vi "WaitPassTacticCheckStateChange.vi"(4 "Tactic index in":i32, 6 "Role ofRobotThat\nmake the pass":T1=enum."PassKicker", 8 "error in (no error)":errorcluster, 9 "Robot in":refnum<class "Robot.lvclass">, 10 "Game":refnum<class "Game.lvclass">, 11 "WaitPassTactic in":refnum<class "WaitPassTactic.lvclass">) -> (0 "error out":errorcluster, 2 "States":enum16{"State 0", "State 1", "State 2", "Exit"}(ring), 3 "WaitPassTactic out":refnum<class "WaitPassTactic.lvclass">)   [LabVIEW 2023, in "WaitPassTactic.lvclass"]
uses:
  WaitPassTactic.lvclass
  Game_class/Game.lvclass
  Robot_class/roles.ctl
  Robot_class/Robot.lvclass
  Game_class/Game.lvclass/Game.ctl
  Team_class/Team.lvclass/Team.ctl
  Robot_class/Robot.lvclass/Robot.ctl
  Robot_class/Read role.vi
  Game_class/Read OffensiveTeam.vi
  Game_class/Read Utilities.lvclass.vi
  Game_class/Read BallRef.vi
  Team_class/Read RobotRef.vi
  Ally_class/Ally.lvclass
  Utilities_class/Utilities.lvclass
  Ball_class/Ball.lvclass
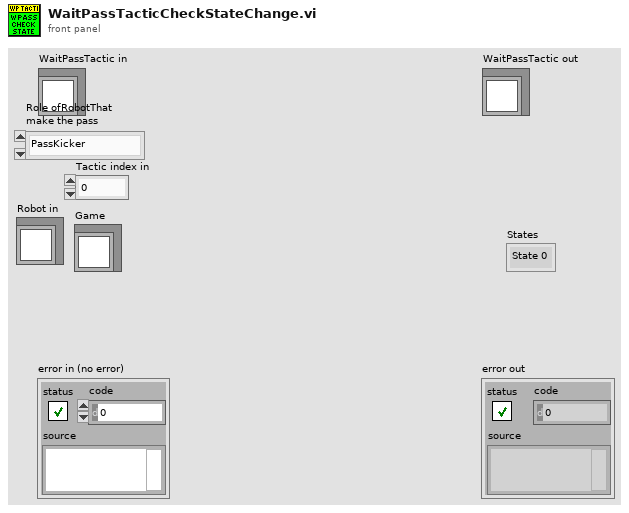
[diagram p1: front panel]
types:
  T1 = typedef "roles.ctl" = enum16{"BallChallengerAttackerVSS", "NormalAttackerVSS", "AttackerAimGoalVSS", "DefenderAreaVSS", "KeeperVSS", "Tabler", "TableFinalizer", "PrepareRollToPassRoller", "PrepareRollToPassReceiver", "SimplePassRoll", "SimplePassRollReceiver", "PenaltyDefense", "PreparePassReceiver 2", "PreparePassReceiver 1", "PassObserver", "Timeout", "Goto", "ZigZag", "None", "BallOutOfField", "DefenderArea", "Duelist", "AttackerStop", "FollowAttacker", "KeeperRole", "KickPenalty", "AttackerAimGoal", "AttackerBlock", "Marker", "Halt", "Shoot", "PassKicker", "PassReceiver", "TestRole", "PenaltyAttacker"}
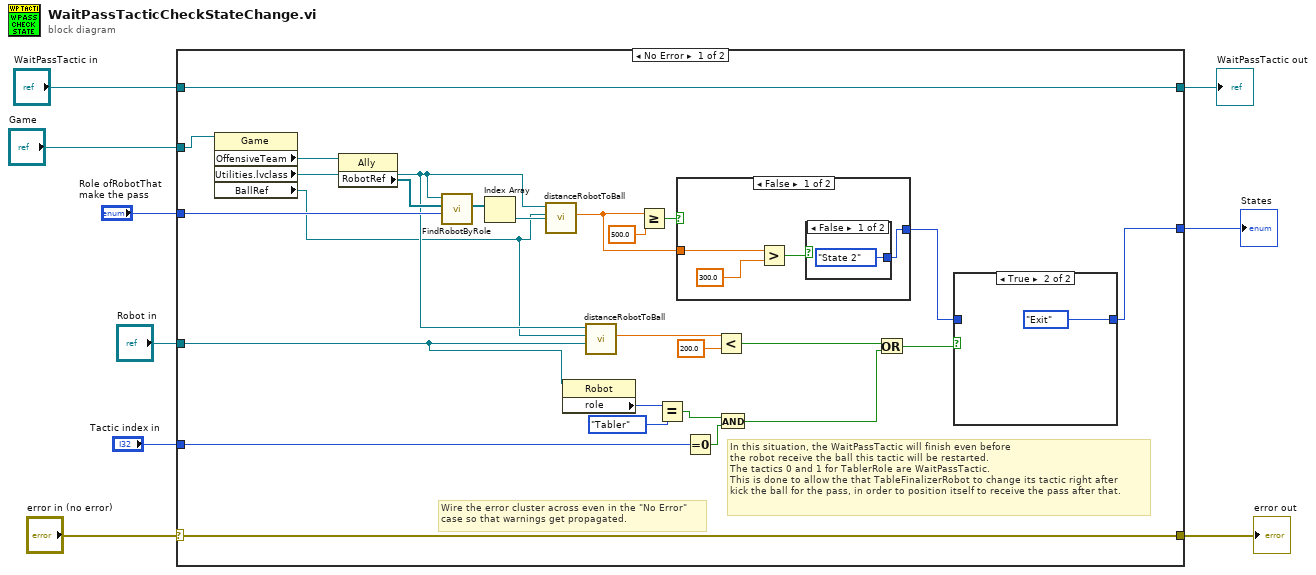
[diagram p0: block diagram]
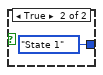
[diagram p3: hidden frame]
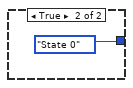
[diagram p4: hidden frame]
diagram:
  n1 = case shown="No Error" "error in (no error)" {
    selector: "error in (no error)" -> [w35 w46]
    tunnel: [w35 w46] -> w8
    tunnel: [w34 w45] -> w6
    tunnel: "WaitPassTactic in" -> [w34 w45]
    tunnel: [w22 _] -> w4
    tunnel: "Game" -> [w26 _]
    tunnel: "Role ofRobotThat\nmake the pass" -> [w21 _]
    tunnel: "Robot in" -> [w17 _]
    tunnel: "Tactic index in" -> [w12 _]
    frame No Error {
      # "In this situation, the WaitPassTactic will finish even before\nthe robot receive the ball this tactic will be restarted. \nThe tactics 0 and 1 for TablerRole are WaitPassTactic.\nThis is done to allow the that TableFinalizerRobot to change its tactic right after\nkick the ball for the pass, in order to position itself to receive the pass after that."
      # "Wire the error cluster across even in the \"No Error\"\ncase so that warnings get propagated."
      n2 = property class="Game"(reference=w26) -> ("OffensiveTeam"=w33:refnum<class "Ally.lvclass">, "Utilities.lvclass"=w20:refnum<class "Utilities.lvclass">, "BallRef"=w10:refnum<class "Ball.lvclass">)  [unwired: 1 in, 2 out]
      n3 = property class="Ally"(reference=w33) -> ("RobotRef"=w27:refnum<class "Robot.lvclass">[])  [unwired: 1 in, 2 out]
      n4 = call "FindRobotByRole.vi"("role"=w21, "RobotRef"=w27, "Utilities in"=w20) -> ("Robots"=w30:refnum<class "Robot.lvclass">[])  [unwired: 6 in, 2 out]
      n5 = Index Array(array=w30) -> (element=w29:refnum<class "Robot.lvclass">)  [unwired: 1 in]
      n6 = call "distanceRobotToBall.vi"("Robot"=w29, "Ball"=w10, "Utilities in"=w20) -> ("Distance Robot To Ball"=w28:dbl)  [unwired: 6 in, 2 out]
      n7 = property class="Robot"(reference=w17) -> ("role"=w16:T1)  [unwired: 1 in, 2 out]
      n8 = call "distanceRobotToBall.vi"("Robot"=w17, "Ball"=w10, "Utilities in"=w20) -> ("Distance Robot To Ball"=w25:dbl)  [unwired: 6 in, 2 out]
      n9 = Greater Or Equal?(x=w28, y=500.0) -> (x >= y?=w31:bool)
      n10 = Equal?(x=w16, y=roles."Tabler") -> (x = y?=w14:bool)
      n11 = case shown="False" w31 {
        tunnel: [w39 enum16{"State 0", "State 1", "State 2", "Exit"}."State 0" ("States")] -> w23
        tunnel: w28 -> [w38 _]
        frame False {
          n12 = Greater?(x=w38, y=300.0) -> (0:w40:bool)
          n13 = case shown="False" w40 {
            tunnel: [enum16{"State 0", "State 1", "State 2", "Exit"}."State 2" ("States") enum16{"State 0", "State 1", "State 2", "Exit"}."State 1" ("States")] -> w39
            frame False {
            }
            frame True {
            }
          }
        }
        frame True {
        }
      }
      n14 = Equal To 0?(x=w12) -> (x = 0?=w13:bool)
      n15 = Less?(x=w25, y=200.0) -> (x < y?=w18:bool)
      n16 = And(x=w14, y=w13) -> (x .and. y?=w11:bool)
      n17 = Or(x=w18, y=w11) -> (x .or. y?=w19:bool)
      n18 = case shown="True" w19 {
        tunnel: w23 -> [w36 _]
        tunnel: [w36 enum16{"State 0", "State 1", "State 2", "Exit"}."Exit" ("States")] -> w22
        frame False {
        }
        frame True {
        }
      }
    }
    frame Error {
    }
  }
  "error out" <- w8
  "WaitPassTactic out" <- w6
  "States" <- w4
